vi "Setup Path Group.vi"(0 "Path Group in":refnum<class "Path Group.lvclass">, 11 "error in":errorcluster) -> (4 "Path Group out":refnum<class "Path Group.lvclass">, 6 "Path Callbacks Reference":refnum<vi>[](array[refnum]), 15 "error out":errorcluster)   [LabVIEW 2023, in "RFFixtureCharact.Public.lvlib"]
uses:
  RFFixtureCharact.Public.lvlib
  Common/Base Classes/Path Group/Path Group.lvclass
  Common/Base Classes/Path/Path.lvclass
  Common/RFCalAndFixtureCharact.Common.lvlib
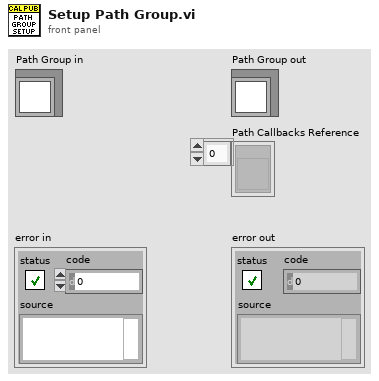
[diagram p1: front panel]
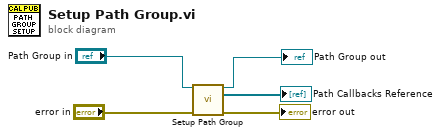
[diagram p0: block diagram]
diagram:
  n1 = call "Setup Path Group.vi"("Path Group in"="Path Group in", "error in"="error in") -> ("Path Group out"=→"Path Group out":refnum<class "Path Group.lvclass">, "Path Callbacks Reference"=→"Path Callbacks Reference":refnum<vi>[], "error out"=→"error out":errorcluster)  [unwired: 11 in]
